vi "Initialize.vi"(8 "error in (no error)":errorcluster, 9 "Baud Rate":u32(ring)=9600 items=["9600"=9600, "38400"=38400, "57600"=57600, "19200"=19200], 10 "Simulate":bool, 11 "VISA resource name":refnum<visa-resource-name>) -> (0 "error out":errorcluster, 3 "VISA resource name out":refnum<visa-resource-name>)   [LabVIEW 2012, in "FEM-03.lvlib"]
doc: "Establishes communication with the instrument and optionally performs an instrument identification query and/or an instrument reset. It also places the instrument in a default state needed for other instrument driver operations. Therefore, call this VI before calling other instrument driver VIs for this instrument. Generally, you need to call the Initialize VI only once at the beginning of an application."
uses:
  FEM-03.lvlib
panel:
  # "(c) 2007 <Enter Company Name Here>.  ALL RIGHTS RESERVED."
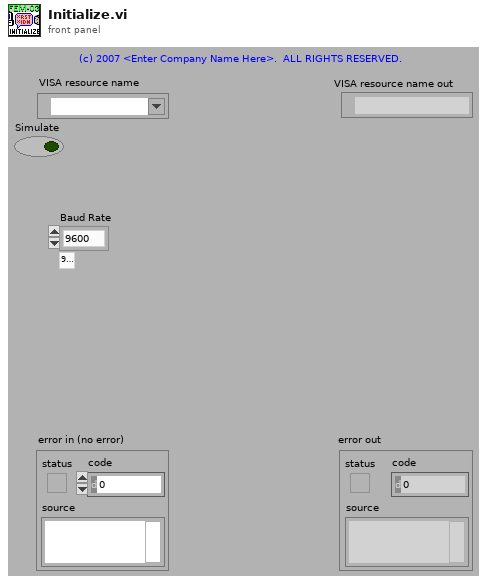
[diagram p1: front panel]
types:
  T1 = cluster{"Baud Rate":u32, "Parity":u16, "Data Bits":u16, "Stop Bits":u16, "Flow Control":u16}
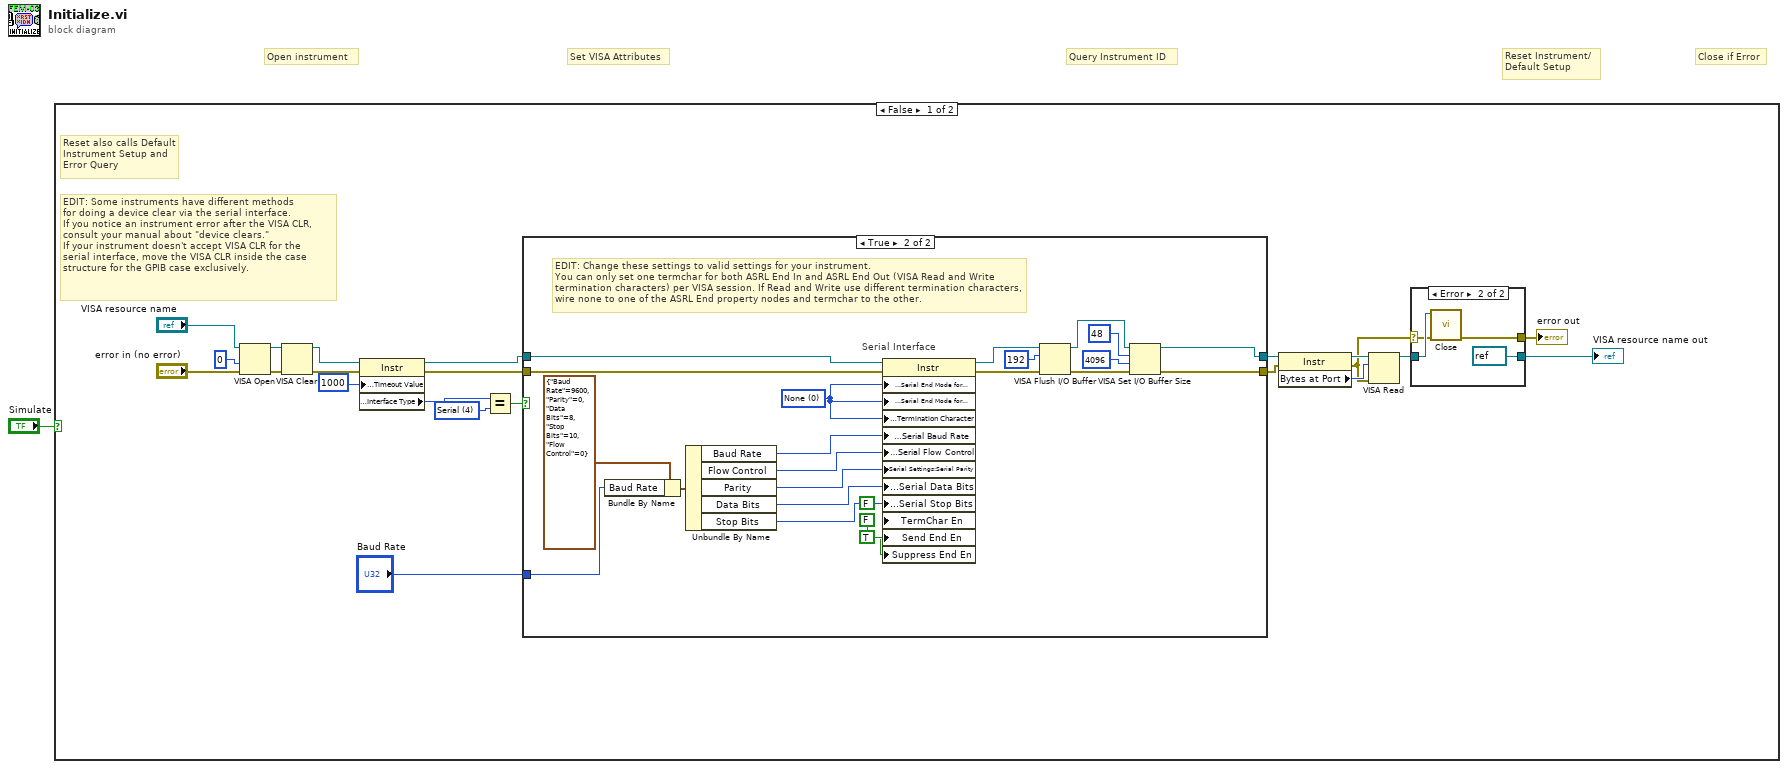
[diagram p0: block diagram]
diagram:
  # "Set VISA Attributes"
  # "Close if Error"
  # "Query Instrument ID"
  # "Reset Instrument/\nDefault Setup"
  # "Open instrument"
  n1 = case shown="False" "Simulate" {
    frame False {
      w16 = u16 4 items=["GPIB"=1, "VXI"=2, "GPIB-VXI"=3, "Serial"=4, "PXI"=5, "TCPIP"=6, "USB"=7] ("Interface Information:Interface Type")
      # "Reset also calls Default Instrument Setup and Error Query"
      # "EDIT: Some instruments have different methods\nfor doing a device clear via the serial interface.  \nIf you notice an instrument error after the VISA CLR,\nconsult your manual about \"device clears.\"  \nIf your instrument doesn't accept VISA CLR for the\nserial interface, move the VISA CLR inside the case \nstructure for the GPIB case exclusively."
      n2 = VISA Open(access mode=u32 0, error in (no error)="error in (no error)", VISA resource name="VISA resource name") -> (VISA resource name=w14:refnum<visa-resource-name>, error out=w13:errorcluster)  [unwired: 2 in]
      n3 = VISA Clear(VISA resource name=w14, error in (no error)=w13) -> (VISA resource name out=w12:refnum<visa-resource-name>, error out=w11:errorcluster)
      n4 = property class="Instr"(reference=w12, error in=w11, "General Settings:Timeout Value"=u32 1000) -> (reference out=w19:refnum<visa-resource-name>, error out=w18:errorcluster, "Interface Information:Interface Type"=w21:u16)
      n5 = Equal?(x=w21, y=w16) -> (x = y?=w17:bool)
      n6 = case shown="True" w17 {
        tunnel: [w24 w45] -> w7
        tunnel: [w25 w42] -> w4
        tunnel: w19 -> [w24 w47]
        tunnel: w18 -> [w25 w48]
        tunnel: "Baud Rate" -> [_ w26]
        frame False {
          # "EDIT: Remove interfaces not\nsupported by your instrument."
          # "GPIB, TCP/IP, and USB Interface"
        }
        frame True {
          w28 = u16 0 items=["None", "LastBit", "TermChar"] ("Serial Settings:Serial End Mode for Reads")
          # "EDIT: Change these settings to valid settings for your instrument.\nYou can only set one termchar for both ASRL End In and ASRL End Out (VISA Read and Write termination characters) per VISA session. If Read and Write use different termination characters, wire none to one of the ASRL End property nodes and termchar to the other."
          # "Serial Interface"
          n7 = Bundle By Name(cluster=T1 {"Baud Rate"=9600, "Parity"=0, "Data Bits"=8, "Stop Bits"=10, "Flow Control"=0} ("Serial Configuration"), "Baud Rate"=w26) -> (w27:T1)
          n8 = Unbundle By Name(w27) -> ("Baud Rate"=w37:u32, "Flow Control"=w33:u16, "Parity"=w35:u16, "Data Bits"=w36:u16, "Stop Bits"=w32:u16)
          n9 = property class="Instr"(reference=w47, error in=w48, "Serial Settings:Serial End Mode for Reads"=w28, "Serial Settings:Serial End Mode for Writes"=w28, "Message Based Settings:Termination Character"=w28, "Serial Settings:Serial Baud Rate"=w37, "Serial Settings:Serial Flow Control"=w33, "Serial Settings:Serial Parity"=w35, "Serial Settings:Serial Data Bits"=w36, "Serial Settings:Serial Stop Bits"=w32, "TermChar En"=FALSE ("Message Based Settings:Termination Character Enable"), "Send End En"=FALSE ("Message Based Settings:Send End Enable"), "Suppress End En"=TRUE ("Message Based Settings:Suppress End Enable")) -> (reference out=w41:refnum<visa-resource-name>, error out=w44:errorcluster)
          n10 = VISA Flush I/O Buffer(VISA resource name=w41, mask (16)=u16 192, error in (no error)=w44) -> (VISA resource name out=w46:refnum<visa-resource-name>, error out=w43:errorcluster)
          n11 = VISA Set I/O Buffer Size(VISA resource name=w46, mask (16)=u16 48, size (4096)=u32 4096 ("size (0)"), error in (no error)=w43) -> (VISA resource name out=w45:refnum<visa-resource-name>, error out=w42:errorcluster)
        }
      }
      n12 = property class="Instr"(reference=w7, error in=w4) -> (reference out=w6:refnum<visa-resource-name>, error out=w3:errorcluster, "Bytes at Port"=w5:u32)
      n13 = VISA Read(VISA resource name=w6, byte count=w5, error in (no error)=w3) -> (VISA resource name out=w8:refnum<visa-resource-name>)  [unwired: 3 out]
      n14 = case shown="Error" w3 {
        selector: w3 -> [w49 w52]
        tunnel: w8 -> [w50 w53]
        tunnel: [w50 refnum<visa-resource-name> refnum ("VISA resource name out")] -> w10
        tunnel: [w49 w54] -> w9
        frame No Error {
        }
        frame Error {
          n15 = call "Close.vi"("error in (no error)"=w52, "VISA resource name"=w53) -> ("error out"=w54:errorcluster)  [unwired: 9 in]
        }
      }
      "VISA resource name out" <- w10
      "error out" <- w9
    }
    frame True {
    }
  }
